vi "Even or ODD VI.vi"() -> ()   [LabVIEW 2020]
panel:
  out "Even Or Odd":string
  out "Boolean":bool
  in  "Numeric":dbl
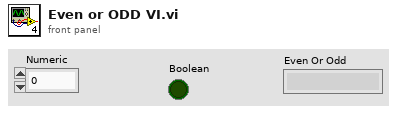
[diagram p1: front panel]
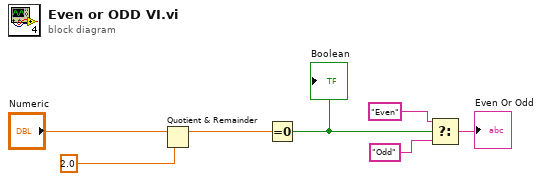
[diagram p0: block diagram]
diagram:
  n1 = Quotient & Remainder(x="Numeric", y=2.0) -> (x-y*floor(x/y)=w5:dbl)  [unwired: 1 out]
  n2 = Equal To 0?(x=w5) -> (x = 0?=w4:bool)
  "Boolean" <- w4
  n3 = Select(t="Even", s=w4, f="Odd") -> (s? t:f=→"Even Or Odd":string)
